vi "Stop SubComponent.vi"(5 "Component ID":u8, 7 "FPGA Interface":refnum<class "FPGA Interface.lvclass">, 8 "error in (no error)":errorcluster, 11 "Bus Controller in":refnum<class "Bus Controller.lvclass">) -> (0 "error out":errorcluster, 3 "Bus Controller out":refnum<class "Bus Controller.lvclass">)   [LabVIEW 2020, in "BCI-1553 API.lvlib" / "Bus Controller.lvclass"]
doc: "Disables this Bus Controller, stops this Bus Controller, and re-enables this Bus Controller shortly after."
uses:
  Bus Controller.lvclass
  Dependencies/FPGA Interface/FPGA Interface.lvclass
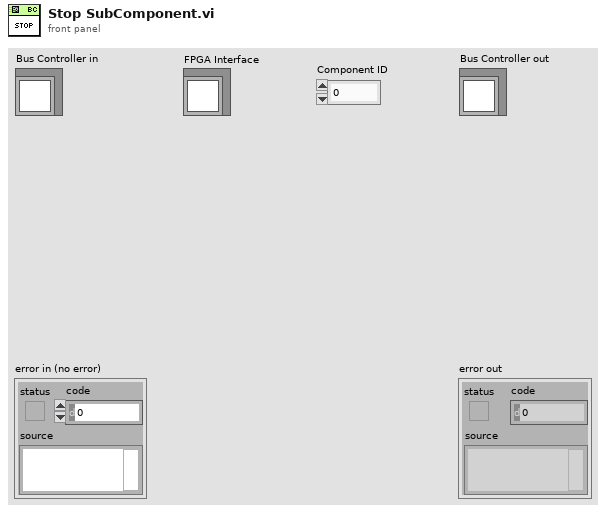
[diagram p1: front panel]
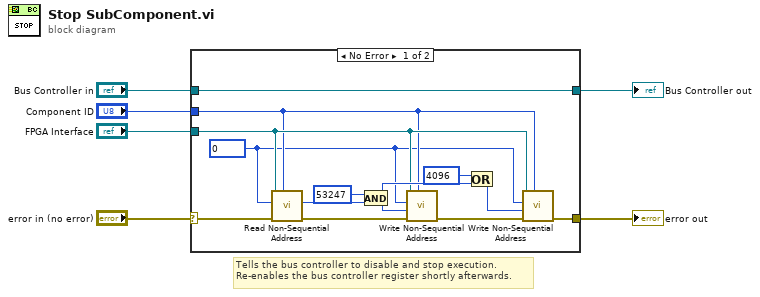
[diagram p0: block diagram]
diagram:
  # "Tells the bus controller to disable and stop execution.\nRe-enables the bus controller register shortly afterwards."
  n1 = case shown="No Error" "error in (no error)" {
    selector: "error in (no error)" -> [w19 w21]
    tunnel: [w7 w21] -> w2
    tunnel: "Bus Controller in" -> [w8 w20]
    tunnel: "FPGA Interface" -> [w13 _]
    tunnel: "Component ID" -> [w12 _]
    tunnel: [w8 w20] -> w1
    frame No Error {
      w9 = u16 0 ("Address")
      n2 = call-dynamic "Read Non-Sequential Address.vi"("Target IC (1-8)"=w12, "error in (no error)"=w19, "Address"=w9, "FPGA Interface in"=w13) -> ("error out"=w18:errorcluster, "Data"=w16:u16)  [unwired: 6 in]
      n3 = And(x=u16 53247 ("Address"), y=w16) -> (x .and. y?=w14:u16)
      n4 = call-dynamic "Write Non-Sequential Address.vi"("Target IC (1-8)"=w12, "error in (no error)"=w18, "Data"=w14, "Address"=w9, "FPGA Interface in"=w13) -> ("error out"=w11:errorcluster)  [unwired: 6 in]
      n5 = Or(x=u16 4096 ("Address"), y=w14) -> (x .or. y?=w10:u16)
      n6 = call-dynamic "Write Non-Sequential Address.vi"("Target IC (1-8)"=w12, "error in (no error)"=w11, "Data"=w10, "Address"=w9, "FPGA Interface in"=w13) -> ("error out"=w7:errorcluster)  [unwired: 6 in]
    }
    frame Error {
    }
  }
  "error out" <- w2
  "Bus Controller out" <- w1
